vi "Actor Core.vi"(8 "error in":errorcluster, 11 "Stepper3D in":refnum<class "Stepper3D.lvclass">) -> (0 "error out":errorcluster, 3 "Actor  out":refnum<class "Actor.lvclass">)   [LabVIEW 2014, in "Stepper3D.lvclass"]
uses:
  Stepper3D.lvclass
  <vilib>/Utility/config.llb/NI_LVConfig.lvlib
  <vilib>/Utility/error.llb/DialogType.ctl
  Libs/array.lib/Array.lvlib
  Libs/stepper3D.lib/stepper3D.lvlib
  Libs/stepper3D.lib/Enums/BoundaryStatus.ctl
  <vilib>/Utility/config.llb/Read Key (Double).vi
  <vilib>/Utility/config.llb/Write Key (Double).vi
  Framework/Interfaces/Viewable Actor/Viewable Actor.lvclass
  Framework/Interfaces/Observable Actor/Observable Actor.lvclass
  Framework/Hardware/ParameterDevice/ParameterDevice.lvclass
  Stepper3D Messages/Set Conversion Table Msg/Set Conversion Table Msg.lvclass
  <vilib>/ActorFramework/Actor/Actor.lvclass
panel:
  in  "St3:DoSteps":bool
  in  "St2:DoSteps":bool
  out "WL:Real Value":dbl=450.0
  out "Stop":bool=TRUE
  out "St3:Right":bool
  out "St3:Left":bool
  out "St2:Right":bool
  out "St2:Left":bool
  out "St1:Right":bool
  out "St1:Left":bool
  in  "Speed":string="300"
  in  "UI:LoadConversionTables":bool
  in  "Conversion 3":path=path "C:/Users/219-PC/Dropbox/МФД/Alexandr Bogomolov/Кумарин 47/Эталон.txt"
  in  "Conversion 2":path=path "C:/Users/219-PC/Dropbox/МФД/Alexandr Bogomolov/Кумарин 47/Эталон.txt"
  in  "Conversion 1":path=path "C:/Users/219-PC/Dropbox/МФД/Alexandr Bogomolov/Кумарин 47/Кумарин 120.txt"
  out "WL:WLToStepper3":dbl[][](array[numeric])
  out "WL:WLToStepper2":dbl[][](array[numeric])=[[115.0, 0.0], [135.0, 0.0]]
  out "WL:WLToStepper1":dbl[][](array[numeric])
  in  "WL:NewValue":dbl=450.0
  in  "WL:Stop":bool
  in  "WL:SetValue":bool
  out "App:RefreshLED":bool
  in  "App:RefreshRate":u32=1000 caption="Refresh every"
  in  "App:Refresh":bool
  in  "App:Disconnect":bool
  in  "App:Connect":bool
  in  "St3:SetPos":bool
  in  "St2:SetPos":bool
  in  "St1:SetPos":bool
  in  "St:Stop":bool
  in  "St3:Steps":dbl
  in  "St3:NewPosition":dbl=2605.0
  out "St3:Position":dbl=2903.0
  in  "St2:Steps":dbl
  in  "St2:NewPosition":dbl=-2500.0
  out "St2:Position":dbl=-2500.0
  in  "St1:DoSteps":bool
  in  "St1:Steps":dbl
  in  "St1:NewPosition":dbl=-57680.0
  out "St1:Position":dbl=-57680.0
  in  "App:ResourceName":refnum<visa-resource-name>="COM8"
  # "ms."
  # "BOUNDARY"
  # "FUNCTIONS"
  # "POSITION"
  # "NEW POSITION"
  # "STEPS"
  # "Решетка"
  # "Фабри-Перо"
  # "Кристалл"
  # "Длина волны"
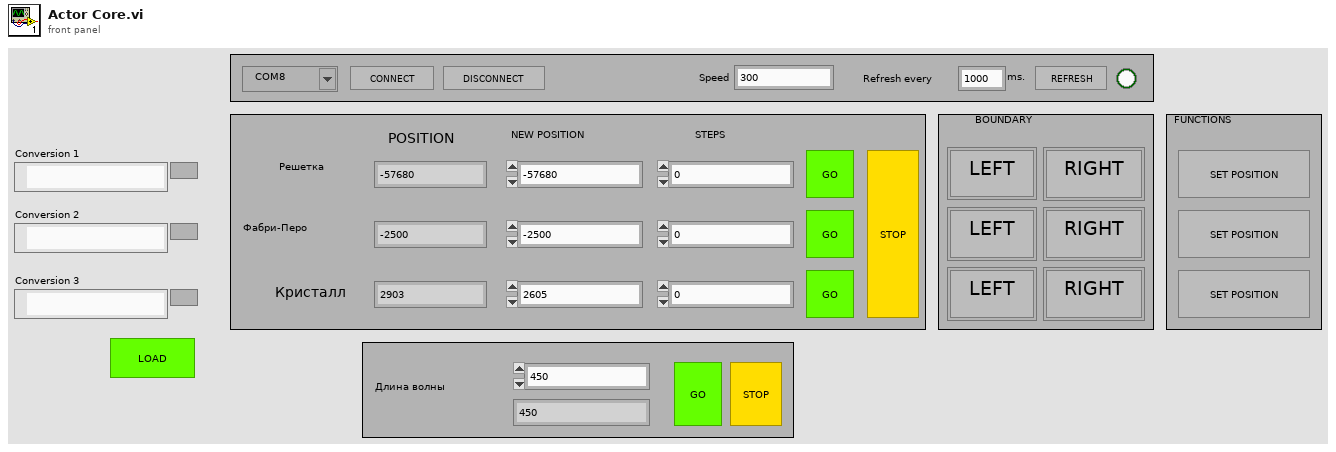
[diagram p1: front panel]
types:
  T1 = typedef "Observable Actor.lvlib/Observable Actor.lvclass/Observer.ctl" = refnum<queue>
  T2 = cluster{"steps":i32, "position":i32, "left":bool, "right":bool, "isRunning":bool, "stepper":u32}
  T3 = enum32{"invalid app kind", "Development System", "Run Time System", "Student Edition", "Embedded LabVIEW", "Evaluation", "Custom"}
  T4 = typedef "stepper3D.lvlib/BoundaryStatus.ctl" = enum16{"NO BOUNDARY", "OUT OF LEFT", "OUT OF RIGHT"}
  T5 = cluster{"Core":cluster{"Current VI Reference":refnum<vi>, "Close Panel on Exit?":bool}, "VISA resource":refnum<visa-resource-name>, "App:RefreshRate":u32, "isConnected":bool, "appended path":path}
  T6 = typedef "DialogType.ctl" = u16
  T7 = cluster{"Current VI Reference":refnum<vi>, "Close Panel on Exit?":bool}
  T8 = typedef "NI_LVConfig.lvlib/Config Data RefNum.ctl" = refnum<k1>
  T9 = enum8{"Enabled", "Disabled", "Disabled and Grayed Out"}
  T10 = typedef "stepper3D.lvlib/CurrentStatus.ctl" = cluster{"desired":dbl[], "current":dbl[], "boundaries":T4[], "is running":bool}
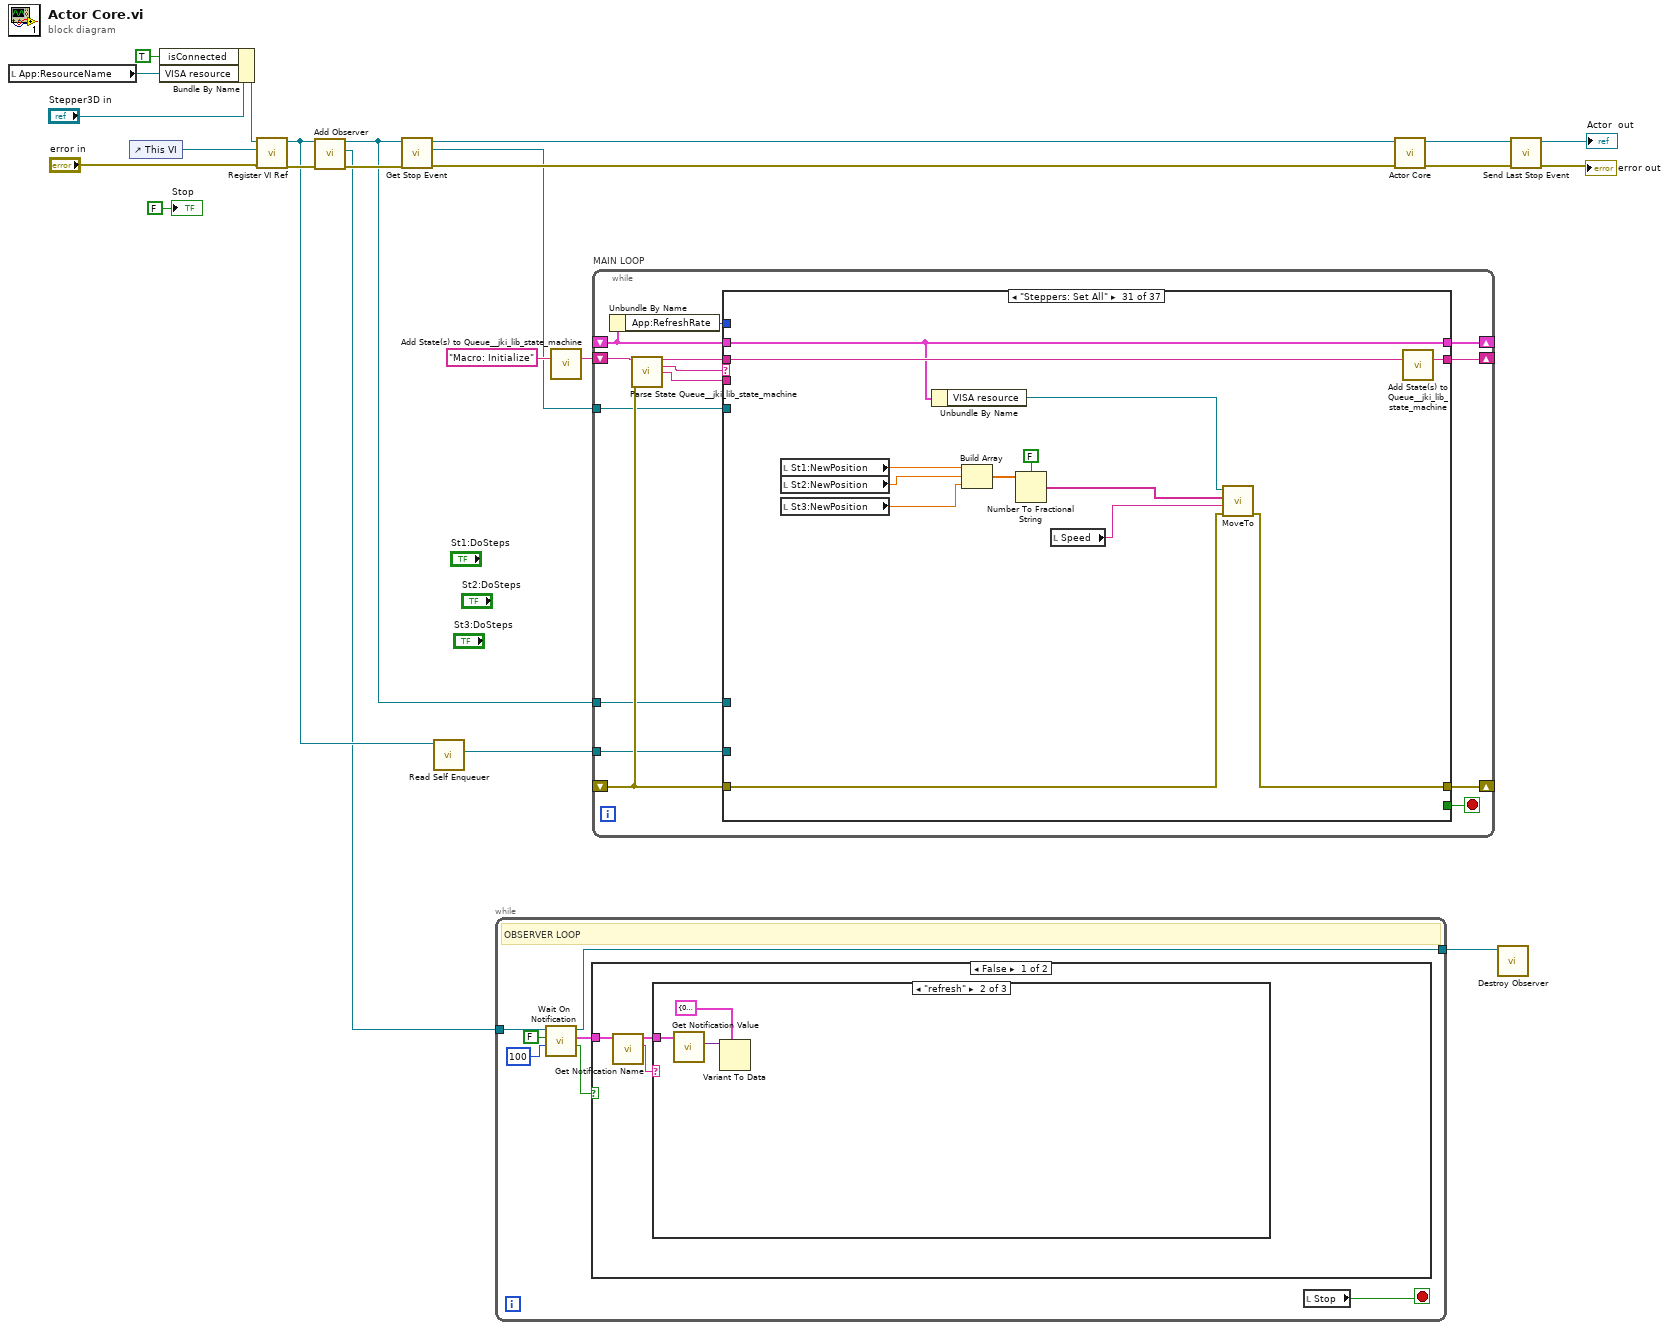
[diagram p0: block diagram]
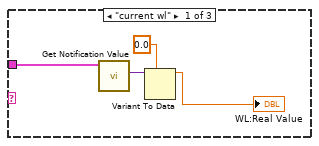
[diagram p2: hidden frame]
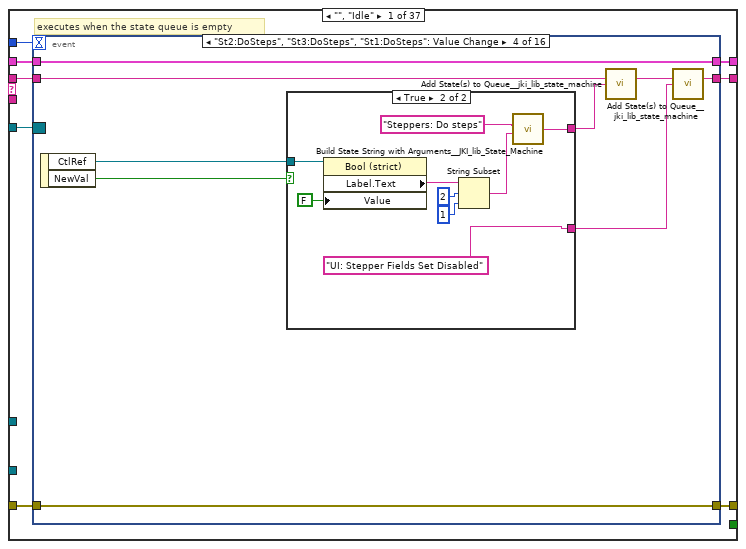
[diagram p5: hidden frame]
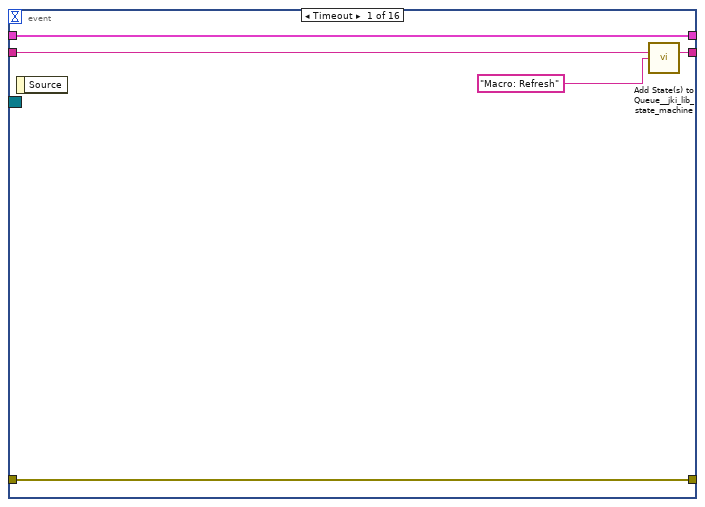
[diagram p6: hidden frame]
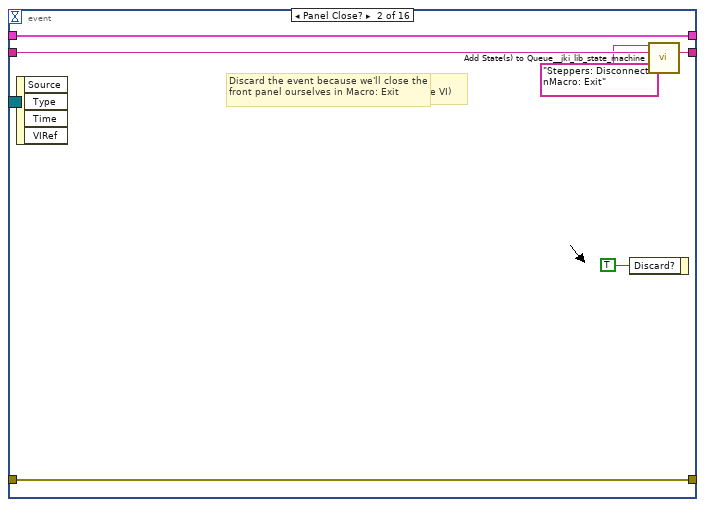
[diagram p7: hidden frame]
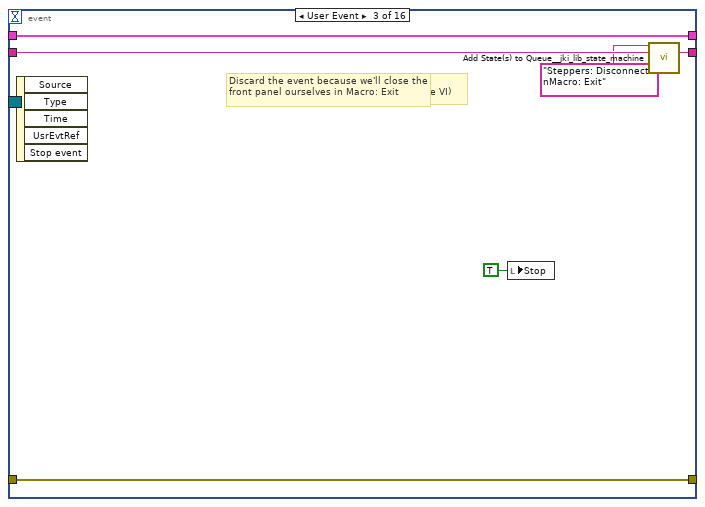
[diagram p8: hidden frame]
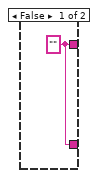
[diagram p9: hidden frame]
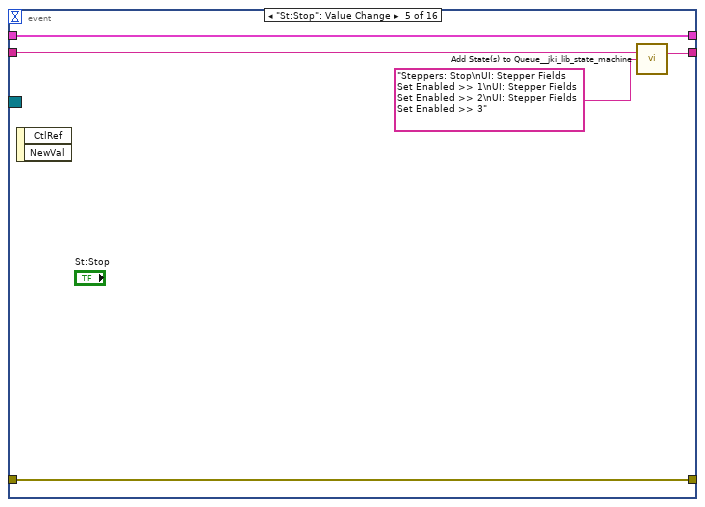
[diagram p10: hidden frame]
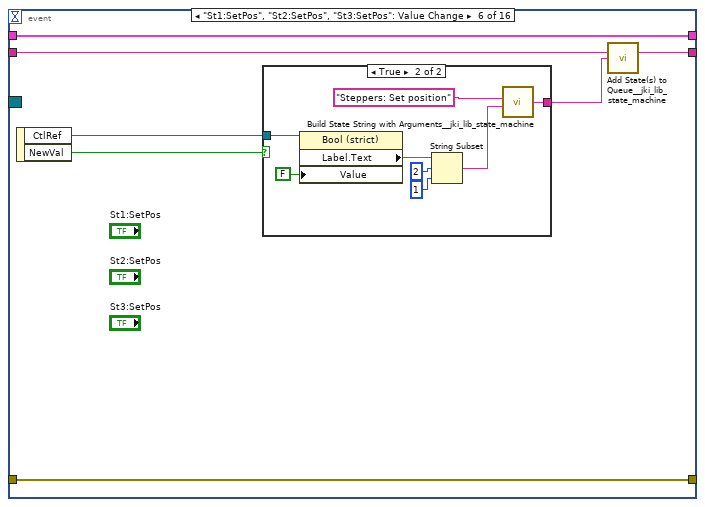
[diagram p11: hidden frame]
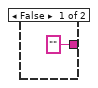
[diagram p12: hidden frame]
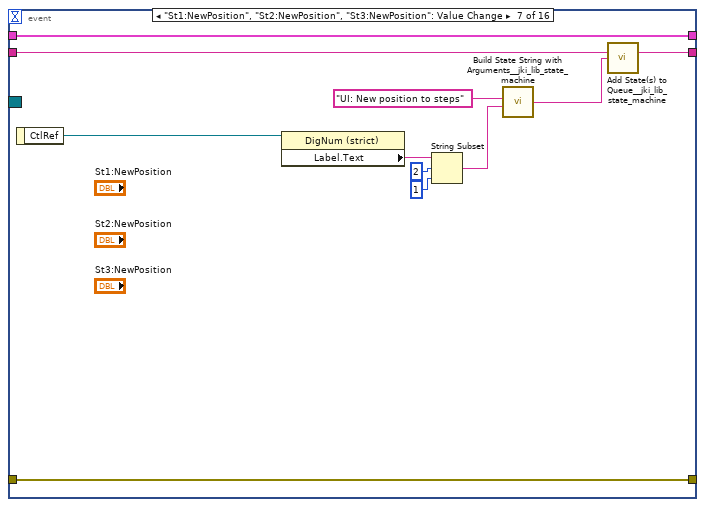
[diagram p13: hidden frame]
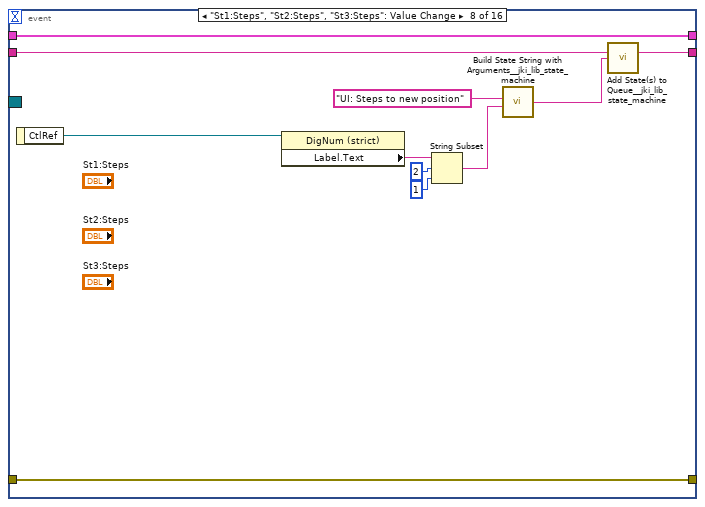
[diagram p14: hidden frame]
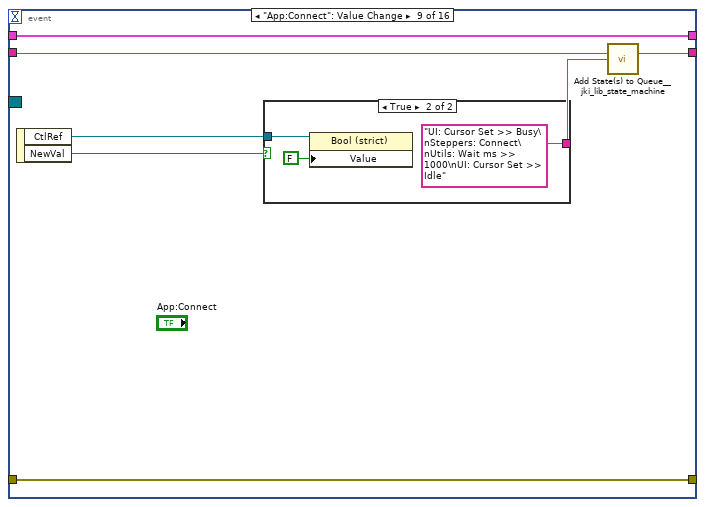
[diagram p15: hidden frame]
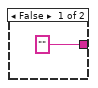
[diagram p16: hidden frame]
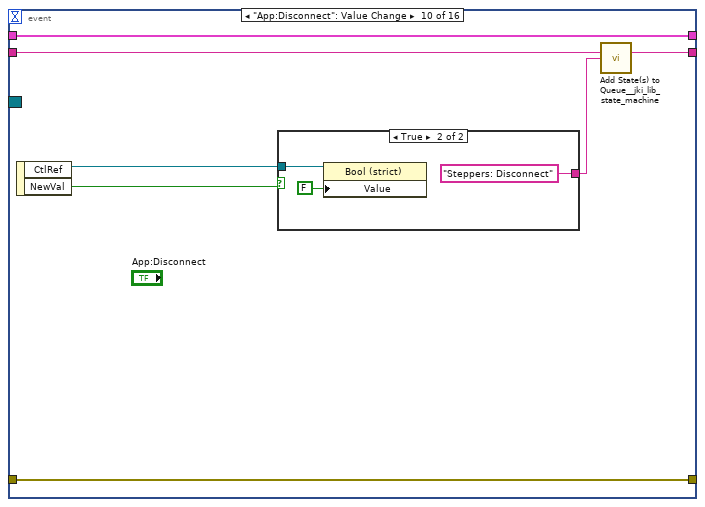
[diagram p17: hidden frame]
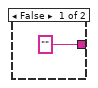
[diagram p18: hidden frame]
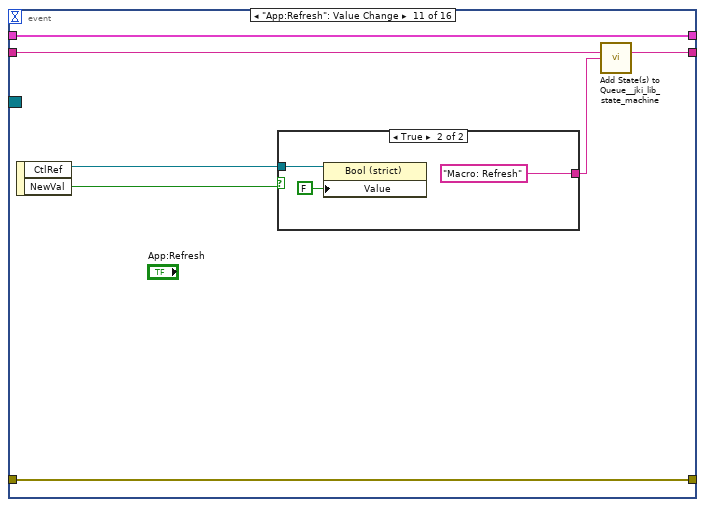
[diagram p19: hidden frame]
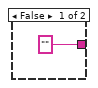
[diagram p20: hidden frame]
diagram:
  n1 = local read "App:ResourceName"() -> (w9:refnum<visa-resource-name>)
  n2 = control-ref of="This VI"() -> (w19:refnum<vi>)
  n3 = Bundle By Name(cluster="Stepper3D in", "isConnected"=TRUE, "VISA resource"=w9) -> (w11:refnum<class "Stepper3D.lvclass">)
  n4 = call "Register VI Ref.vi"("error in (no error)"="error in", "VI ref"=w19, "Viewable Actor in"=w11) -> ("error out"=w20:errorcluster, "Viewable Actor out"=w7:refnum<class "Stepper3D.lvclass">)  [unwired: 7 in]
  n5 = call-dynamic "Add Observer.vi"("error in (no error)"=w20, "Observable Actor in"=w7) -> ("error out"=w21:errorcluster, "new observer"=w2:T1, "Observable Actor out"=w1:refnum<class "Stepper3D.lvclass">)  [unwired: 7 in]
  n6 = call-dynamic "Get Stop Event.vi"("error in (no error)"=w21, "Observable Actor in"=w1) -> ("error out"=w14:errorcluster, "Events"=w8:refnum<event-registration>, "Observable Actor out"=w15:refnum<class "Stepper3D.lvclass">)  [unwired: 7 in]
  n7 = call <vilib>:"Read Self Enqueuer.vi"("Actor"=w7) -> ("Self Enqueuer"=w6:refnum<class "Message Enqueuer.lvclass">)  [unwired: 10 in]
  n8 = while {
    tunnel: w2 -> [w27]
    tunnel: [w26] -> w4
    stop <- w30 stop-if-true
    # "OBSERVER LOOP"
    n9 = call "Wait On Notification.vi"("timeout in ms (-1)"=100, "ignore previous (F)"=FALSE, "observer in"=w27) -> ("timed out?"=w24:bool, "notification"=w25:cluster{"value":variant, "name":string}, "observer out"=w26:T1)  [unwired: 5 in, 1 out]
    n10 = case shown="False" w24 {
      tunnel: w25 -> [w33 _]
      frame False {
        n11 = call "Get Notification Name.vi"("notification in"=w33) -> ("name"=w31:string, "notification out"=w32:cluster{"value":variant, "name":string})  [unwired: 9 in]
        n12 = case shown="\"refresh\"" w31 {
          tunnel: w32 -> [w35 w39 _]
          frame "current wl" {
            n13 = call "Get Notification Value.vi"("notification in"=w35) -> ("data"=w37:variant)  [unwired: 7 in, 1 out]
            n14 = Variant To Data(type=0.0 ("Current value"), Variant=w37) -> (data=→"WL:Real Value":dbl)  [unwired: 1 in, 1 out]
          }
          frame "refresh" {
            n15 = call "Get Notification Value.vi"("notification in"=w39) -> ("data"=w40:variant)  [unwired: 7 in, 1 out]
            n16 = Variant To Data(type=T2 {"steps"=0, "position"=0, "left"=FALSE, "right"=FALSE, "isRunning"=FALSE, "stepper"=0} ("input cluster"), Variant=w40) -> ()  [unwired: 1 in, 2 out]
          }
          frame Default {
          }
        }
      }
      frame True {
      }
    }
    n17 = local read "Stop"() -> (w30:bool)
  }
  n18 = call <vilib>:"Add State(s) to Queue__jki_lib_state_machine.vi"("State(s) in (\"\")"="Macro: Initialize") -> ("States Out"=w23:string)  [unwired: 14 in]
  n19 = while "MAIN LOOP" {
    shift-right: [w48] -> _
    shift-left: _ -> [w44]
    shift-right: [w51] -> _
    shift-left: _ -> [w47]
    shift-right: [w50] -> _
    shift-left: w23 -> [w52]
    tunnel: w8 -> [w43]
    tunnel: w6 -> [w42]
    tunnel: w1 -> [w41]
    stop <- w49 stop-if-true
    n20 = Unbundle By Name(w44) -> ("App:RefreshRate"=w45:u32)
    n21 = call <vilib>:"Parse State Queue__jki_lib_state_machine.vi"("State Queue"=w52, "Error In (no error)"=w47) -> ("Remaining States"=w54:string, "Current State"=w46:string, "Arguments"=w53:string)  [unwired: 11 in]
    n22 = case shown="\"Steppers: Set All\"" w46 {
      selector: w46 -> [_ _ w215 _ _ _ _ _ _ _ _ _ _ _ _ _ _ _ _ _ _ _ _ _ _ _ _ _ _ _ _ _ _ _ _ _ _]
      tunnel: w54 -> [w62 w214 w219 w237 w244 w249 w253 w268 w279 w298 w320 w326 w330 w335 w340 w345 w347 w366 w369 w385 w386 w394 w399 w404 w410 w422 w426 w434 w441 w460 w477 w494 w505 w508 w576 w581 w588]
      tunnel: w53 -> [_ _ _ _ _ _ _ _ _ _ _ _ _ _ _ _ w346 _ w370 _ w389 _ _ _ _ _ _ _ _ w450 _ w490 _ _ _ _ w584]
      tunnel: w44 -> [w60 w211 w217 w228 w241 w247 w250 w265 _ w296 w317 w322 w327 w332 w337 w343 w349 w368 w372 w383 w390 w395 w396 w401 w407 w419 w423 w437 w440 w458 w475 w491 w503 w513 w577 w578 w585]
      tunnel: [w59 w212 w221 w234 errorcluster {"status"=FALSE, "code"=0, "source"=""} ("error out") w246 w251 w266 w276 w280 w318 w323 w328 w333 w338 w342 w348 w367 w371 w382 w388 w393 w397 w402 w408 w420 w424 w427 w442 w455 w472 w489 w500 w510 w572 w579 w586] -> w51
      tunnel: w47 -> [w58 w212 w220 w234 w240 w246 w251 w266 w276 w281 w318 w321 w328 w333 w338 w342 w348 w367 w371 w382 w388 w393 w397 w402 w408 w420 w424 w428 w443 w456 w473 w488 w501 w511 w573 w579 w586]
      tunnel: [w61 w213 w218 w236 w243 w248 w252 w267 w278 w297 w319 w325 w329 w334 w339 w344 w347 w366 w369 w384 w386 w394 w398 w403 w409 w421 w425 w435 w441 w459 w476 w493 w504 w507 w575 w580 w587] -> w50
      tunnel: [_ _ _ _ _ TRUE _ _ _ _ _ _ _ _ _ _ _ _ _ _ _ _ _ _ _ _ _ _ _ _ _ _ _ _ _ _ _] -> w49
      tunnel: [w57 w211 w217 w235 w241 w247 w250 w265 w277 w296 w317 w322 w327 w332 w337 w343 w349 w368 w372 w383 w390 w395 w396 w401 w407 w419 w423 w436 w439 w458 w475 w491 w503 w513 w577 w578 w585] -> w48
      tunnel: w45 -> [w56 _ _ _ _ _ _ _ _ _ _ _ _ _ _ _ _ _ _ _ _ _ _ _ _ _ _ _ _ _ _ _ _ _ _ _ _]
      tunnel: w43 -> [w55 _ _ _ _ _ _ _ _ _ _ _ _ _ _ _ _ _ _ _ _ _ _ _ _ _ _ _ _ _ _ _ _ _ _ _ _]
      tunnel: w42 -> [_ _ _ _ _ _ _ w257 _ _ _ _ _ _ _ _ _ _ _ _ _ _ _ _ _ _ _ _ _ _ _ _ _ _ _ _ _]
      tunnel: w41 -> [_ _ _ _ _ _ _ _ _ _ _ _ _ _ _ _ _ _ _ _ _ _ _ _ _ _ _ _ _ _ _ _ _ _ w574 _ _]
      frame "", "Idle" {
        # "executes when the state queue is empty"
        n23 = event shown="[3] \"St2:DoSteps\", \"St3:DoSteps\", \"St1:DoSteps\": Value Change" {
          selector: w55 -> [_ _ _ _ _ _ _ _ _ _ _ _ _ _ _ _]
          dyn-events: _ -> [_ _ _ _ _ _ _ _ _ _ _ _ _ _ _ _]
          timeout: w56 -> [_ _ _ _ _ _ _ _ _ _ _ _ _ _ _ _]
          tunnel: w62 -> [w67 w73 w79 w84 w100 w106 w127 w138 w145 w155 w166 w180 w185 w191 w199 w207]
          tunnel: [w66 w72 w78 w82 w101 w105 w126 w137 w146 w156 w167 w181 w186 w192 w200 w208] -> w61
          tunnel: w60 -> [w64 w70 w76 w87 w103 w109 w129 w140 w147 w159 w170 w177 w183 w189 w197 w205]
          tunnel: [w65 w71 w77 w86 w102 w108 w128 w139 w148 w153 w164 w178 w184 w190 w198 w206] -> w59
          tunnel: w58 -> [w65 w71 w77 w86 w102 w108 w128 w139 w148 w153 w164 w178 w184 w190 w198 w206]
          tunnel: [w64 w70 w76 w87 w103 w109 w129 w140 w147 w159 w170 w176 w183 w189 w197 w205] -> w57
          event Timeout {
            n24 = event-data() -> ()  [unwired: 1 in, 1 out]
            n25 = call <vilib>:"Add State(s) to Queue__jki_lib_state_machine.vi"("State(s) in (\"\")"=w67, "State(s) at Back (\"\")"="Macro: Refresh") -> ("States Out"=w66:string)  [unwired: 13 in]
          }
          event Panel Close? {
            # "Discard the event because we'll close the front panel ourselves in Macro: Exit"
            # "Close Panel button (pressed) Event\n(this executes Macro: Exit to terminate the VI)"
            n26 = event-data() -> ()  [unwired: 1 in, 4 out]
            n27 = event-data("Discard?"=TRUE) -> ()  [unwired: 1 in, 1 out]
            n28 = call <vilib>:"Add State(s) to Queue__jki_lib_state_machine.vi"("State(s) in Front (\"\")"="Steppers: Disconnect\nMacro: Exit", "State(s) in (\"\")"=w73) -> ("States Out"=w72:string)  [unwired: 13 in]
          }
          event User Event {
            # "Discard the event because we'll close the front panel ourselves in Macro: Exit"
            # "Close Panel button (pressed) Event\n(this executes Macro: Exit to terminate the VI)"
            n29 = event-data() -> ()  [unwired: 1 in, 5 out]
            n30 = local write "Stop"(TRUE ("Stop")) -> ()
            n31 = call <vilib>:"Add State(s) to Queue__jki_lib_state_machine.vi"("State(s) in Front (\"\")"="Steppers: Disconnect\nMacro: Exit", "State(s) in (\"\")"=w79) -> ("States Out"=w78:string)  [unwired: 13 in]
          }
          event "St2:DoSteps", "St3:DoSteps", "St1:DoSteps": Value Change {
            n32 = event-data() -> ("CtlRef"=w88:refnum<vi>, "NewVal"=w85:bool)  [unwired: 1 in]
            n33 = case shown="True" w85 {
              tunnel: w88 -> [_ w98]
              tunnel: [w89 w94] -> w83
              tunnel: [w89 "UI: Stepper Fields Set Disabled" ("State")] -> w80
              frame False {
                w89 = "" ("State with Arguments")
              }
              frame True {
                n34 = property class="Bool (strict)"(reference=w98, "Value"=FALSE) -> ("Label.Text"=w91:string)  [unwired: 1 in, 2 out]
                n35 = String Subset(string=w91, offset (0)=2, length (rest)=1 ("length (rest)")) -> (substring=w90:string)
                n36 = call <vilib>:"Build State String with Arguments__JKI_lib_State_Machine.vi"("Arguments (\"\")"=w90, "State"="Steppers: Do steps") -> ("State with Arguments"=w94:string)  [unwired: 4 in]
              }
            }
            n37 = call <vilib>:"Add State(s) to Queue__jki_lib_state_machine.vi"("State(s) in (\"\")"=w84, "State(s) at Back (\"\")"=w83) -> ("States Out"=w81:string)  [unwired: 13 in]
            n38 = call <vilib>:"Add State(s) to Queue__jki_lib_state_machine.vi"("State(s) in (\"\")"=w81, "State(s) at Back (\"\")"=w80) -> ("States Out"=w82:string)  [unwired: 13 in]
          }
          event "St:Stop": Value Change {
            n39 = event-data() -> ()  [unwired: 1 in, 2 out]
            n40 = call <vilib>:"Add State(s) to Queue__jki_lib_state_machine.vi"("State(s) in (\"\")"=w100, "State(s) at Back (\"\")"="Steppers: Stop\nUI: Stepper Fields Set Enabled >> 1\nUI: Stepper Fields Set Enabled >> 2\nUI: Stepper Fields Set Enabled >> 3" ("State")) -> ("States Out"=w101:string)  [unwired: 13 in]
          }
          event "St1:SetPos", "St2:SetPos", "St3:SetPos": Value Change {
            n41 = event-data() -> ("CtlRef"=w110:refnum<vi>, "NewVal"=w107:bool)  [unwired: 1 in]
            n42 = case shown="True" w107 {
              tunnel: w110 -> [_ w119]
              tunnel: ["" ("State with Arguments") w113] -> w104
              frame False {
              }
              frame True {
                n43 = property class="Bool (strict)"(reference=w119, "Value"=FALSE) -> ("Label.Text"=w116:string)  [unwired: 1 in, 2 out]
                n44 = String Subset(string=w116, offset (0)=2, length (rest)=1 ("length (rest)")) -> (substring=w114:string)
                n45 = call <vilib>:"Build State String with Arguments__jki_lib_state_machine.vi"("Arguments (\"\")"=w114, "State"="Steppers: Set position") -> ("State with Arguments"=w113:string)  [unwired: 4 in]
              }
            }
            n46 = call <vilib>:"Add State(s) to Queue__jki_lib_state_machine.vi"("State(s) in (\"\")"=w106, "State(s) at Back (\"\")"=w104) -> ("States Out"=w105:string)  [unwired: 13 in]
          }
          event "St1:NewPosition", "St2:NewPosition", "St3:NewPosition": Value Change {
            n47 = event-data() -> ("CtlRef"=w130:refnum<vi>)  [unwired: 1 in]
            n48 = property class="DigNum (strict)"(reference=w130) -> ("Label.Text"=w122:string)  [unwired: 1 in, 2 out]
            n49 = String Subset(string=w122, offset (0)=2, length (rest)=1 ("length (rest)")) -> (substring=w120:string)
            n50 = call <vilib>:"Build State String with Arguments__jki_lib_state_machine.vi"("Arguments (\"\")"=w120, "State"="UI: New position to steps") -> ("State with Arguments"=w125:string)  [unwired: 4 in]
            n51 = call <vilib>:"Add State(s) to Queue__jki_lib_state_machine.vi"("State(s) in (\"\")"=w127, "State(s) at Back (\"\")"=w125) -> ("States Out"=w126:string)  [unwired: 13 in]
          }
          event "St1:Steps", "St2:Steps", "St3:Steps": Value Change {
            n52 = event-data() -> ("CtlRef"=w141:refnum<vi>)  [unwired: 1 in]
            n53 = property class="DigNum (strict)"(reference=w141) -> ("Label.Text"=w133:string)  [unwired: 1 in, 2 out]
            n54 = String Subset(string=w133, offset (0)=2, length (rest)=1 ("length (rest)")) -> (substring=w131:string)
            n55 = call <vilib>:"Build State String with Arguments__jki_lib_state_machine.vi"("Arguments (\"\")"=w131, "State"="UI: Steps to new position") -> ("State with Arguments"=w136:string)  [unwired: 4 in]
            n56 = call <vilib>:"Add State(s) to Queue__jki_lib_state_machine.vi"("State(s) in (\"\")"=w138, "State(s) at Back (\"\")"=w136) -> ("States Out"=w137:string)  [unwired: 13 in]
          }
          event "App:Connect": Value Change {
            n57 = event-data() -> ("CtlRef"=w144:refnum<vi>, "NewVal"=w143:bool)  [unwired: 1 in]
            n58 = case shown="True" w143 {
              tunnel: w144 -> [_ w152]
              tunnel: ["" "UI: Cursor Set >> Busy\nSteppers: Connect\nUtils: Wait ms >> 1000\nUI: Cursor Set >> Idle"] -> w142
              frame False {
              }
              frame True {
                n59 = property class="Bool (strict)"(reference=w152, "Value"=FALSE) -> ()  [unwired: 1 in, 2 out]
              }
            }
            n60 = call <vilib>:"Add State(s) to Queue__jki_lib_state_machine.vi"("State(s) in (\"\")"=w145, "State(s) at Back (\"\")"=w142) -> ("States Out"=w146:string)  [unwired: 13 in]
          }
          event "App:Disconnect": Value Change {
            n61 = event-data() -> ("CtlRef"=w158:refnum<vi>, "NewVal"=w157:bool)  [unwired: 1 in]
            n62 = case shown="True" w157 {
              tunnel: w158 -> [_ w163]
              tunnel: ["" "Steppers: Disconnect"] -> w154
              frame False {
              }
              frame True {
                n63 = property class="Bool (strict)"(reference=w163, "Value"=FALSE) -> ()  [unwired: 1 in, 2 out]
              }
            }
            n64 = call <vilib>:"Add State(s) to Queue__jki_lib_state_machine.vi"("State(s) in (\"\")"=w155, "State(s) at Back (\"\")"=w154) -> ("States Out"=w156:string)  [unwired: 13 in]
          }
          event "App:Refresh": Value Change {
            n65 = event-data() -> ("CtlRef"=w169:refnum<vi>, "NewVal"=w168:bool)  [unwired: 1 in]
            n66 = case shown="True" w168 {
              tunnel: w169 -> [_ w174]
              tunnel: ["" "Macro: Refresh"] -> w165
              frame False {
              }
              frame True {
                n67 = property class="Bool (strict)"(reference=w174, "Value"=FALSE) -> ()  [unwired: 1 in, 2 out]
              }
            }
            n68 = call <vilib>:"Add State(s) to Queue__jki_lib_state_machine.vi"("State(s) in (\"\")"=w166, "State(s) at Back (\"\")"=w165) -> ("States Out"=w167:string)  [unwired: 13 in]
          }
          event "App:RefreshRate": Value Change {
            n69 = event-data() -> ()  [unwired: 1 in, 1 out]
            n70 = Bundle By Name(cluster=w177, "App:RefreshRate"="App:RefreshRate") -> (w176:T5)
            n71 = call <vilib>:"Add State(s) to Queue__jki_lib_state_machine.vi"("State(s) in (\"\")"=w180, "State(s) at Back (\"\")"="Steppers: Set refresh rate") -> ("States Out"=w181:string)  [unwired: 13 in]
          }
          event "WL:NewValue": Value Change {
            n72 = event-data() -> ()  [unwired: 1 in, 6 out]
            n73 = call <vilib>:"Add State(s) to Queue__jki_lib_state_machine.vi"("State(s) in (\"\")"=w185, "State(s) at Back (\"\")"="UI: New WL to positions" ("State(s) at Back (\"\")")) -> ("States Out"=w186:string)  [unwired: 13 in]
          }
          event "WL:SetValue": Value Change {
            n74 = event-data() -> ("NewVal"=w188:bool)  [unwired: 1 in]
            n75 = case shown="False" w188 {
              tunnel: ["" "Steppers: Set All"] -> w187
              frame False {
              }
              frame True {
                n76 = property on="WL:SetValue" class="Bool (strict)"("Value"=FALSE ("WL:SetValue")) -> ()  [unwired: 2 in, 2 out]
              }
            }
            n77 = call <vilib>:"Add State(s) to Queue__jki_lib_state_machine.vi"("State(s) in (\"\")"=w191, "State(s) at Back (\"\")"=w187) -> ("States Out"=w192:string)  [unwired: 13 in]
          }
          event "WL:Stop": Value Change {
            n78 = event-data() -> ("NewVal"=w196:bool)  [unwired: 1 in]
            n79 = case shown="True" w196 {
              frame False {
              }
              frame True {
                n80 = property on="WL:Stop" class="Bool (strict)"("Value"=FALSE ("WL:Stop")) -> ()  [unwired: 2 in, 2 out]
                n81 = property on="St:Stop" class="Bool (strict)"("Val(Sgnl)"=TRUE) -> ()  [unwired: 2 in, 2 out]
              }
            }
            n82 = call <vilib>:"Add State(s) to Queue__jki_lib_state_machine.vi"("State(s) in (\"\")"=w199) -> ("States Out"=w200:string)  [unwired: 14 in]
          }
          event "UI:LoadConversionTables": Value Change {
            n83 = event-data() -> ("NewVal"=w204:bool)  [unwired: 1 in]
            n84 = case shown="True" w204 {
              tunnel: [_ "Data: Load Conversion Files"] -> w203
              frame False {
              }
              frame True {
                n85 = property on="UI:LoadConversionTables" class="Bool (strict)"("Value"=FALSE) -> ()  [unwired: 2 in, 2 out]
              }
            }
            n86 = call <vilib>:"Add State(s) to Queue__jki_lib_state_machine.vi"("State(s) in (\"\")"=w207, "State(s) at Back (\"\")"=w203) -> ("States Out"=w208:string)  [unwired: 13 in]
          }
        }
      }
      frame "---------- Core ----------" {
        # "Do not put any code in this frame.\n(it is a separator no-op)"
        n87 = call <vilib>:"Add State(s) to Queue__jki_lib_state_machine.vi"("State(s) in (\"\")"=w214) -> ("States Out"=w213:string)  [unwired: 14 in]
      }
      frame Default {
        w224 = 42 items=["No error", "Argument error", "Memory is full", "Out of zone", "End of file", "File already open", "Generic file I/O error", "File not found", "File permission error", "Disk is full", "Duplicate path", "Too many files open", "System feature not enabled", "Resource file not found", "Cannot add resource", "Resource not found", "Image not found", "Image memory error", "Pen does not exist", "Config type invalid", "Config token not found", "Config parse error", "Config memory error", "Bad external code format", "Bad external code offset", "External code not present", "Null window", "Destroy window error", "Null menu", "Print aborted", "Bad print record", "Print driver error", "Windows error during printing", "Memory error during printing", "Print dialog error", "Generic print error", "Invalid device refnum", "Device not found", "Device parameter error", "Device unit error", "Cannot open device", "Device call aborted", "Generic error", "Cancelled by user", "Object ID too low", "Object ID too high", "Object not in heap", "Unknown heap", "Unknown object (invalid DefProc)", "Unknown object (DefProc not in table)", "Message out of range", "Invalid (null) method", "Unknown message", "Manager call not supported", "Bad address", "Network operation in progress", "Network operation timed out", "Connection is busy", "Network attribute not supported", "Network error", "Address in use", "System out of memory", "Connection aborted", "Connection refused", "Not connected", "Already connected", "Connection closed", "Initialization error (interapplication manager)", "Bad occurrence", "Wait on unbound occurrence handler", "Occurrence queue overflow", "Datalog type conflict", "Unused", "Unrecognized type (interapplication manager)", "Memory corrupt", "Failed to make temporary DLL", "Old CIN version", "Drag socket not found", "Failed to load drop-object", "Failed to register OLE object", "Failed to release OLE object", "Format specifier type mismatch", "Unknown format specifier", "Too few format specifiers", "Too many format specifiers", "Scan failed", "Newer CIN version", "Error converting to variant", "Runtime menu error", "Password tampered", "Variant attribute not found", "Incompatible variant data type", "Event data is not available", "Event Store is not present", "Occurrence is not found", "Event Queue is not created", "Event info is not available", "Refnum passed is NULL", "Error retrieving Class GUID", "Error retrieving CoClass GUID", "Error retrieving TypeLib GUID.", "Bad built application magic bytes.", "Specific driver is different from the specific driver associated with the Logical Name.", "There is no session opened to the class driver.", "Max Error", "MAX - Error with config objects", "MAX - Error loading configuration", "MAX - Group not supported"]
        # "Current State"
        # "Handle mistyped state name (developer tool)"
        n88 = Format Into String(format string="Software Exception: Unhandled State \"%s\"." ("message"), error in=w220, w215) -> (resulting string=w223:string, error out=w222:errorcluster)  [unwired: 1 in]
        n89 = call <vilib>:"Error Cluster From Error Code.vi"("show call chain? (False)"=TRUE, "error in (no error)"=w222, "error message (\"\")"=w223, "error code (0)"=w224) -> ("error out"=w221:errorcluster)  [unwired: 5 in]
        n90 = call <vilib>:"Add State(s) to Queue__jki_lib_state_machine.vi"("State(s) in (\"\")"=w219) -> ("States Out"=w218:string)  [unwired: 14 in]
      }
      frame "Initialize Core Data" {
        # "originally closed?"
        # "exe?"
        # "If panel starts closed or is an EXE, then close it when we exit"
        n91 = property class="VI"() -> ("Front Panel.Open"=w233:bool)  [unwired: 2 in, 2 out]
        n92 = property class="App"() -> ("App.Kind"=w232:T3)  [unwired: 2 in, 2 out]
        n93 = control-ref of="Current VI Reference"() -> (w226:refnum<vi>)
        n94 = Not(x=w233) -> (.not. x?=w230:bool)
        n95 = Equal?(x=w232, y=T3."Run Time System" ("Application:Kind")) -> (x = y?=w229:bool)
        n96 = Or(x=w230, y=w229) -> (x .or. y?=w227:bool)
        n97 = Bundle By Name(cluster=w228, "Core.Current VI Reference"=w226, "Core.Close Panel on Exit?"=w227) -> (w235:T5)
        n98 = call <vilib>:"Add State(s) to Queue__jki_lib_state_machine.vi"("State(s) in (\"\")"=w237) -> ("States Out"=w236:string)  [unwired: 14 in]
      }
      frame "Error Handler" {
        w238 = T6 2 items=["no dialog", "OK message", "continue or stop message", "OK message + warnings", "continue/stop + warnings"] ("type of dialog (OK msg:1)")
        # "Unhandled Error -- Display it"
        # "Handle any errors here.\nYou can also output any states to clean-up after errors occur"
        # "Clear error"
        n99 = call <vilib>:"General Error Handler.vi"("type of dialog (OK msg:1)"=w238, "error in (no error)"=w240) -> ()  [unwired: 9 in, 5 out]
        n100 = call <vilib>:"Add State(s) to Queue__jki_lib_state_machine.vi"("State(s) in Front (\"\")"="// Post Error States", "State(s) in (\"\")"=w244) -> ("States Out"=w243:string)  [unwired: 13 in]
      }
      frame "Exit" {
        n101 = call <vilib>:"Add State(s) to Queue__jki_lib_state_machine.vi"("State(s) in (\"\")"=w249) -> ("States Out"=w248:string)  [unwired: 14 in]
      }
      frame "---------- Data ----------" {
        # "Do not put any code in this frame.\n(It is a separator no-op. You can make a copy of this frame to create a new Data frame)"
        n102 = call <vilib>:"Add State(s) to Queue__jki_lib_state_machine.vi"("State(s) in (\"\")"=w253) -> ("States Out"=w252:string)  [unwired: 14 in]
      }
      frame "Data: Load Conversion Files" {
        n103 = call "readArrayFromFile.vi"("file"="Conversion 1") -> ("array"=w256:dbl[][])  [unwired: 1 in, 1 out]
        "WL:WLToStepper1" <- w256
        n104 = call "readArrayFromFile.vi"("file"="Conversion 2") -> ("array"=w255:dbl[][])  [unwired: 1 in, 1 out]
        "WL:WLToStepper2" <- w255
        n105 = call "readArrayFromFile.vi"("file"="Conversion 3") -> ("array"=w254:dbl[][])  [unwired: 1 in, 1 out]
        "WL:WLToStepper3" <- w254
        n106 = call "Send Set Conversion Table.vi"("Stepper"=u32 1, "Conversion table"=w256, "Message Enqueuer"=w257) -> ()  [unwired: 7 in, 2 out]
        n107 = call "Send Set Conversion Table.vi"("Stepper"=u32 2, "Conversion table"=w255, "Message Enqueuer"=w257) -> ()  [unwired: 7 in, 2 out]
        n108 = call "Send Set Conversion Table.vi"("Stepper"=u32 3, "Conversion table"=w254, "Message Enqueuer"=w257) -> ()  [unwired: 7 in, 2 out]
        n109 = call <vilib>:"Add State(s) to Queue__jki_lib_state_machine.vi"("State(s) in (\"\")"=w268, "State(s) at Back (\"\")"="UI: New WL to positions" ("State(s) at Back (\"\")")) -> ("States Out"=w267:string)  [unwired: 13 in]
      }
      frame "Data: Initialize" {
        w273 = FALSE  # isConnected
        w274 = refnum<visa-resource-name> refnum  # VISA resource
        w275 = T7 {"Current VI Reference"=refnum, "Close Panel on Exit?"=FALSE}  # Core
        n110 = local read "App:RefreshRate"() -> (w272:u32)
        n111 = call <vilib>:"Application Directory.vi"() -> ("Application Directory"=w271:path)
        n112 = Build Path(base path=w271, name or relative path="steppers.config") -> (appended path=w269:path)
        n113 = Bundle("Core"=w275, "VISA resource"=w274, "App:RefreshRate"=w272, "isConnected"=w273, "appended path"=w269) -> (w277:T5)  [unwired: 1 in]
        n114 = call <vilib>:"Add State(s) to Queue__jki_lib_state_machine.vi"("State(s) in (\"\")"=w279) -> ("States Out"=w278:string)  [unwired: 14 in]
      }
      frame "Data: Read Config" {
        n115 = Unbundle By Name(w296) -> ("appended path"=w283:path)
        n116 = call <vilib>:"Open Config Data.vi"("error in (no error)"=w281, "configuration file path"=w283) -> ("error out"=w280:errorcluster, "refnum"=w282:T8)  [unwired: 7 in, 1 out]
        n117 = call-poly <vilib>:"Read Key.vi"("section"="current values", "key"="wavelength", "refnum"=w282) -> ("value"=w287:dbl)  [unwired: 5 in, 3 out]
        n118 = call-poly <vilib>:"Read Key.vi"("section"="current values", "key"="stepper1", "refnum"=w282) -> ("value"=w286:dbl)  [unwired: 5 in, 3 out]
        n119 = call-poly <vilib>:"Read Key.vi"("section"="current values", "key"="stepper2", "refnum"=w282) -> ("value"=w285:dbl)  [unwired: 5 in, 3 out]
        n120 = call-poly <vilib>:"Read Key.vi"("section"="current values", "key"="stepper3", "refnum"=w282) -> ("value"=w284:dbl)  [unwired: 5 in, 3 out]
        n121 = local write "WL:NewValue"(w287) -> ()
        n122 = local write "St1:NewPosition"(w286) -> ()
        n123 = local write "St2:NewPosition"(w285) -> ()
        n124 = local write "St3:NewPosition"(w284) -> ()
        n125 = call <vilib>:"Add State(s) to Queue__jki_lib_state_machine.vi"("State(s) in (\"\")"=w298) -> ("States Out"=w297:string)  [unwired: 14 in]
      }
      frame "Data: Write Config" {
        n126 = Unbundle By Name(w317) -> ("appended path"=w301:path)
        n127 = local read "St1:Position"() -> (w307:dbl)
        n128 = local read "WL:NewValue"() -> (w308:dbl)
        n129 = local read "St2:Position"() -> (w306:dbl)
        n130 = local read "St3:Position"() -> (w305:dbl)
        n131 = call <vilib>:"Open Config Data.vi"("configuration file path"=w301) -> ("refnum"=w300:T8)  [unwired: 8 in, 2 out]
        n132 = call-poly <vilib>:"Write Key.vi"("section"="current values", "value"=w308, "key"="wavelength", "refnum"=w300) -> ("refnum out"=w304:T8)  [unwired: 5 in, 2 out]
        n133 = call-poly <vilib>:"Write Key.vi"("section"="current values", "value"=w307, "key"="stepper1", "refnum"=w304) -> ("refnum out"=w303:T8)  [unwired: 5 in, 2 out]
        n134 = call-poly <vilib>:"Write Key.vi"("section"="current values", "value"=w306, "key"="stepper2", "refnum"=w303) -> ("refnum out"=w302:T8)  [unwired: 5 in, 2 out]
        n135 = call-poly <vilib>:"Write Key.vi"("section"="current values", "value"=w305, "key"="stepper3", "refnum"=w302) -> ("refnum out"=w299:T8)  [unwired: 5 in, 2 out]
        n136 = call <vilib>:"Close Config Data.vi"("refnum"=w299) -> ()  [unwired: 9 in, 2 out]
        n137 = call <vilib>:"Add State(s) to Queue__jki_lib_state_machine.vi"("State(s) in (\"\")"=w320) -> ("States Out"=w319:string)  [unwired: 14 in]
      }
      frame "Data: Cleanup" {
        n138 = Unbundle By Name(w322) -> ("Core.Current VI Reference"=w324:refnum<vi>)
        n139 = Close Reference(reference=w324, error in (no error)=w321) -> (error out=w323:errorcluster)
        n140 = call <vilib>:"Add State(s) to Queue__jki_lib_state_machine.vi"("State(s) in (\"\")"=w326) -> ("States Out"=w325:string)  [unwired: 14 in]
      }
      frame "---------- UI ----------" {
        # "Do not put any code in this frame.\n(It is a separator no-op. You can make a copy of this frame to create a new UI frame)"
        n141 = call <vilib>:"Add State(s) to Queue__jki_lib_state_machine.vi"("State(s) in (\"\")"=w330) -> ("States Out"=w329:string)  [unwired: 14 in]
      }
      frame "UI: Stepper Fields Set Enabled" {
        w331 = T9."Enabled" ("Disabled")
        # "Set Stepper Fields state .\n(Usage: \"UI: Stepper Fields Set Enabled >> 'Stepper Number'\")"
        n142 = property on="St1:NewPosition" class="DigNum (strict)"("DisabledEnum"=w331) -> ()  [unwired: 2 in, 2 out]
        n143 = property on="St2:NewPosition" class="DigNum (strict)"("DisabledEnum"=w331) -> ()  [unwired: 2 in, 2 out]
        n144 = property on="St1:Steps" class="DigNum (strict)"("DisabledEnum"=w331) -> ()  [unwired: 2 in, 2 out]
        n145 = property on="St2:Steps" class="DigNum (strict)"("DisabledEnum"=w331) -> ()  [unwired: 2 in, 2 out]
        n146 = property on="St3:NewPosition" class="DigNum (strict)"("DisabledEnum"=w331) -> ()  [unwired: 2 in, 2 out]
        n147 = property on="St3:Steps" class="DigNum (strict)"("DisabledEnum"=w331) -> ()  [unwired: 2 in, 2 out]
        n148 = property on="St1:DoSteps" class="Bool (strict)"("DisabledEnum"=w331) -> ()  [unwired: 2 in, 2 out]
        n149 = call <vilib>:"Add State(s) to Queue__jki_lib_state_machine.vi"("State(s) in (\"\")"=w335) -> ("States Out"=w334:string)  [unwired: 14 in]
      }
      frame "UI: Stepper Fields Set Disabled" {
        w336 = T9."Disabled and Grayed Out" ("Disabled")
        # "Set Stepper Fields state .\n(Usage: \"UI: Stepper Fields Set Enabled >> 'Stepper Number'\")"
        n150 = property on="St1:NewPosition" class="DigNum (strict)"("DisabledEnum"=w336) -> ()  [unwired: 2 in, 2 out]
        n151 = property on="St1:Steps" class="DigNum (strict)"("DisabledEnum"=w336) -> ()  [unwired: 2 in, 2 out]
        n152 = property on="St2:NewPosition" class="DigNum (strict)"("DisabledEnum"=w336) -> ()  [unwired: 2 in, 2 out]
        n153 = property on="St2:Steps" class="DigNum (strict)"("DisabledEnum"=w336) -> ()  [unwired: 2 in, 2 out]
        n154 = property on="St3:NewPosition" class="DigNum (strict)"("DisabledEnum"=w336) -> ()  [unwired: 2 in, 2 out]
        n155 = property on="St3:Steps" class="DigNum (strict)"("DisabledEnum"=w336) -> ()  [unwired: 2 in, 2 out]
        n156 = property on="St1:DoSteps" class="Bool (strict)"("DisabledEnum"=w336) -> ()  [unwired: 2 in, 2 out]
        n157 = call <vilib>:"Add State(s) to Queue__jki_lib_state_machine.vi"("State(s) in (\"\")"=w340) -> ("States Out"=w339:string)  [unwired: 14 in]
      }
      frame "UI: Initialize" {
        n158 = call <vilib>:"Add State(s) to Queue__jki_lib_state_machine.vi"("State(s) in Front (\"\")"="UI: Stepper Fields Set Enabled" ("State(s) in Front (\"\")"), "State(s) in (\"\")"=w345) -> ("States Out"=w344:string)  [unwired: 13 in]
      }
      frame "UI: Steps to new position" {
        n159 = case shown="\"3\"" w346 {
          frame "1" {
            n160 = local read "St1:Position"() -> (w352:dbl)
            n161 = local read "St1:Steps"() -> (w351:dbl)
            n162 = Add(x=w352, y=w351) -> (x+y=w350:dbl)
            n163 = local write "St1:NewPosition"(w350) -> ()
          }
          frame "2" {
            n164 = local read "St2:Position"() -> (w355:dbl)
            n165 = local read "St2:Steps"() -> (w354:dbl)
            n166 = Add(x=w355, y=w354) -> (x+y=w353:dbl)
            n167 = local write "St2:NewPosition"(w353) -> ()
          }
          frame "3" {
            n168 = local read "St3:Position"() -> (w358:dbl)
            n169 = local read "St3:Steps"() -> (w357:dbl)
            n170 = Add(x=w358, y=w357) -> (x+y=w356:dbl)
            n171 = local write "St3:NewPosition"(w356) -> ()
          }
          frame Default {
          }
        }
      }
      frame "UI: New WL to positions" {
        n172 = local read "WL:WLToStepper1"() -> (w365:dbl[][])
        n173 = local read "WL:WLToStepper2"() -> (w363:dbl[][])
        n174 = local read "WL:WLToStepper3"() -> (w364:dbl[][])
        n175 = property on="WL:NewValue" class="DigNum (strict)"() -> ("Value"=w359:dbl)  [unwired: 2 in, 2 out]
        n176 = call "GetNearestValue.vi"("Value"=w359, "Array"=w365) -> ("Nearest Value"=w362:dbl)  [unwired: 9 in]
        n177 = call "GetNearestValue.vi"("Value"=w359, "Array"=w363) -> ("Nearest Value"=w361:dbl)  [unwired: 9 in]
        n178 = call "GetNearestValue.vi"("Value"=w359, "Array"=w364) -> ("Nearest Value"=w360:dbl)  [unwired: 9 in]
        n179 = property on="St1:NewPosition" class="DigNum (strict)"("Val(Sgnl)"=w362) -> ()  [unwired: 2 in, 2 out]
        n180 = property on="St2:NewPosition" class="DigNum (strict)"("Val(Sgnl)"=w361) -> ()  [unwired: 2 in, 2 out]
        n181 = property on="St3:NewPosition" class="DigNum (strict)"("Val(Sgnl)"=w360) -> ()  [unwired: 2 in, 2 out]
      }
      frame "UI: New position to steps" {
        n182 = case shown="Default" w370 {
          frame Default {
          }
          frame "1" {
            n183 = local read "St1:NewPosition"() -> (w375:dbl)
            n184 = local read "St1:Position"() -> (w374:dbl)
            n185 = Subtract(x=w375, y=w374) -> (x-y=w373:dbl)
            n186 = local write "St1:Steps"(w373) -> ()
          }
          frame "2" {
            n187 = local read "St2:NewPosition"() -> (w378:dbl)
            n188 = local read "St2:Position"() -> (w377:dbl)
            n189 = Subtract(x=w378, y=w377) -> (x-y=w376:dbl)
            n190 = local write "St2:Steps"(w376) -> ()
          }
          frame "3" {
            n191 = local read "St3:NewPosition"() -> (w381:dbl)
            n192 = local read "St3:Position"() -> (w380:dbl)
            n193 = Subtract(x=w381, y=w380) -> (x-y=w379:dbl)
            n194 = local write "St3:Steps"(w379) -> ()
          }
        }
      }
      frame "UI: Cursor Set" {
        # "Set and Unset Cursor Busy.\n(Usage: \"UI: Cursor Set >> Busy|Idle\")"
        n195 = call <vilib>:"Add State(s) to Queue__jki_lib_state_machine.vi"("State(s) in (\"\")"=w385) -> ("States Out"=w384:string)  [unwired: 14 in]
      }
      frame "UI: RefreshLED Set" {
        # "Argument"
        # "Set and Unset RefreshLED.\n(Usage: \"UI: RefreshLED Set >> On|Off\")"
        n196 = case shown="\"Off\", Default" w389 {
          tunnel: [TRUE FALSE] -> w387
          frame "On" {
          }
          frame "Off", Default {
          }
        }
        "App:RefreshLED" <- w387
      }
      frame "UI: Front Panel State" {
        # "Set Front Panel Open or Closed\n(Usage: \"UI: Front Panel State >> Open|Close\")"
      }
      frame "---------- Macro ----------" {
        # "Do not put any code in this frame.\n(It is a separator no-op. You can make a copy of this frame to create a new Macro frame)"
        n197 = call <vilib>:"Add State(s) to Queue__jki_lib_state_machine.vi"("State(s) in (\"\")"=w399) -> ("States Out"=w398:string)  [unwired: 14 in]
      }
      frame "Macro: Initialize" {
        w400 = "Data: Initialize\nInitialize Core Data\nUI: Initialize\nUI: Front Panel State >> Open\nData: Load Conversion Files\nData: Read Config\nSteppers: Connect"  # Data: Initialize Initialize Core Data UI: Initialize UI: Front Panel State >> Open Data: Load Conversion Files Data: Read Config Steppers: Connect
        # "Initialization Macro\n(This is called once, when the VI starts)"
        n198 = call <vilib>:"Add State(s) to Queue__jki_lib_state_machine.vi"("State(s) in Front (\"\")"=w400, "State(s) in (\"\")"=w404) -> ("States Out"=w403:string)  [unwired: 13 in]
      }
      frame "Macro: Refresh" {
        n199 = Unbundle By Name(w407) -> ("isConnected"=w406:bool)
        n200 = case shown="True" w406 {
          tunnel: ["" "UI: RefreshLED Set >> On\nSteppers: Refresh\nSteppers: Refresh WL\nUI: RefreshLED Set >> Off\nData: Write Config"] -> w405
          frame False {
          }
          frame True {
          }
        }
        n201 = call <vilib>:"Add State(s) to Queue__jki_lib_state_machine.vi"("State(s) in Front (\"\")"=w405, "State(s) in (\"\")"=w410) -> ("States Out"=w409:string)  [unwired: 13 in]
      }
      frame "Macro: Exit" {
        # "Exit Macro\n(This is called once, when the VI exits)"
        n202 = Unbundle By Name(w419) -> ("Core.Close Panel on Exit?"=w418:bool)
        n203 = Select(t="UI: Front Panel State >> Close", s=w418, f="") -> (s? t:f=w415:string)
        n204 = call <vilib>:"Add State(s) to Queue__jki_lib_state_machine.vi"("State(s) in (\"\")"=w415, "State(s) at Back (\"\")"="Steppers: Disconnect\nData: Cleanup\nExit") -> ("States Out"=w413:string)  [unwired: 13 in]
        n205 = call <vilib>:"Add State(s) to Queue__jki_lib_state_machine.vi"("State(s) in Front (\"\")"=w413, "State(s) in (\"\")"=w422) -> ("States Out"=w421:string)  [unwired: 13 in]
      }
      frame "---------- Steppers ----------" {
        # "Template Separator\n(You can make a copy of, or modify, this frame)"
        n206 = call <vilib>:"Add State(s) to Queue__jki_lib_state_machine.vi"("State(s) in (\"\")"=w426) -> ("States Out"=w425:string)  [unwired: 14 in]
      }
      frame "Steppers: Connect" {
        # "Connect to steppers"
        n207 = call "connect.vi"("error in"=w428, "VISA resource name"="App:ResourceName") -> ("error out"=w427:errorcluster, "VISA resource name out"=w430:refnum<visa-resource-name>)
        n208 = Unbundle By Name(w427) -> ("status"=w429:bool)
        n209 = Not(x=w429) -> (.not. x?=w432:bool)
        n210 = Bundle By Name(cluster=w437, "isConnected"=w432, "VISA resource"=w430) -> (w436:T5)
        n211 = call <vilib>:"Add State(s) to Queue__jki_lib_state_machine.vi"("State(s) in Front (\"\")"="Macro: Refresh\nSteppers: Set position >> 1\nSteppers: Set position >> 2\nSteppers: Set position >> 3" ("State(s) at Back (\"\")"), "State(s) in (\"\")"=w434) -> ("States Out"=w435:string)  [unwired: 13 in]
      }
      frame "Steppers: Disconnect" {
        n212 = Unbundle By Name(w440) -> ("VISA resource"=w444:refnum<visa-resource-name>)
        n213 = call "disconnect.vi"("error in"=w443, "VISA resource name"=w444) -> ("error out"=w442:errorcluster)  [unwired: 1 in]
        n214 = Bundle By Name(cluster=w440, "isConnected"=FALSE) -> (w439:T5)
      }
      frame "Steppers: Do steps" {
        w451 = ""
        n215 = case shown="Default" w450 {
          tunnel: [0.0 ("St3:NewPosition") w462 w463 w464] -> w452
          frame Default {
          }
          frame "1" {
            n216 = local read "St1:NewPosition"() -> (w462:dbl)
          }
          frame "2" {
            n217 = local read "St2:NewPosition"() -> (w463:dbl)
          }
          frame "3" {
            n218 = local read "St3:NewPosition"() -> (w464:dbl)
          }
        }
        n219 = Decimal String To Number(string=w450) -> (number=w449:i32)  [unwired: 2 in, 1 out]
        n220 = Decrement(x=w449) -> (x-1=w448:i32)
        n221 = Unbundle By Name(w458) -> ("VISA resource"=w457:refnum<visa-resource-name>)
        n222 = Number To Fractional String(use system decimal point (T)=FALSE, number=w452) -> (F-format string=w447:string)  [unwired: 2 in]
        n223 = Build Array(w451, w451, w451) -> (w446:string[])
        n224 = Insert Into Array(array=w446, index=w448, new element=w447) -> (w445:string[])
        n225 = call "MoveTo.vi"("error in (no error)"=w456, "speed"="Speed", "positions"=w445, "VISA Refnum in"=w457) -> ("error out"=w455:errorcluster)  [unwired: 6 in, 1 out]
        n226 = call <vilib>:"Add State(s) to Queue__jki_lib_state_machine.vi"("State(s) in (\"\")"=w460) -> ("States Out"=w459:string)  [unwired: 14 in]
      }
      frame "Steppers: Set All" {
        n227 = local read "St1:NewPosition"() -> (w470:dbl)
        n228 = local read "St2:NewPosition"() -> (w469:dbl)
        n229 = local read "St3:NewPosition"() -> (w468:dbl)
        n230 = Unbundle By Name(w475) -> ("VISA resource"=w474:refnum<visa-resource-name>)
        n231 = Build Array(w470, w469, w468) -> (w467:dbl[])
        n232 = Number To Fractional String(use system decimal point (T)=FALSE, number=w467) -> (F-format string=w466:string[])  [unwired: 2 in]
        n233 = local read "Speed"() -> (w465:string)
        n234 = call "MoveTo.vi"("error in (no error)"=w473, "speed"=w465, "positions"=w466, "VISA Refnum in"=w474) -> ("error out"=w472:errorcluster)  [unwired: 6 in, 1 out]
        n235 = call <vilib>:"Add State(s) to Queue__jki_lib_state_machine.vi"("State(s) in (\"\")"=w477) -> ("States Out"=w476:string)  [unwired: 14 in]
      }
      frame "Steppers: Set position" {
        w486 = ""
        n236 = case shown="\"1\"" w490 {
          tunnel: [0 ("St3:Steps") w496 w497 w498] -> w480
          frame Default {
          }
          frame "1" {
            n237 = local read "St1:NewPosition"() -> (w496:dbl)
          }
          frame "2" {
            n238 = local read "St2:NewPosition"() -> (w497:dbl)
          }
          frame "3" {
            n239 = local read "St3:NewPosition"() -> (w498:dbl)
          }
        }
        n240 = Decimal String To Number(string=w490, default (0L)=u16 0 ("default (0 I32)")) -> (number=w484:u16)  [unwired: 1 in, 1 out]
        n241 = Decrement(x=w484) -> (x-1=w483:u16)
        n242 = Build Array(w486, w486, w486) -> (w485:string[])
        n243 = Unbundle By Name(w491) -> ("VISA resource"=w487:refnum<visa-resource-name>)
        n244 = Number To Fractional String(use system decimal point (T)=FALSE, number=w480) -> (F-format string=w478:string)  [unwired: 2 in]
        n245 = Replace Array Subset(array=w485, new element=w478, index=w483) -> (w482:string[])
        n246 = call "SetPosition.vi"("error in (no error)"=w488, "positions"=w482, "VISA Refnum in"=w487) -> ("error out"=w489:errorcluster)  [unwired: 7 in, 1 out]
        n247 = call <vilib>:"Add State(s) to Queue__jki_lib_state_machine.vi"("State(s) in (\"\")"=w494, "State(s) at Back (\"\")"="Data: Write Config" ("State(s) at Back (\"\")")) -> ("States Out"=w493:string)  [unwired: 13 in]
      }
      frame "Steppers: Stop" {
        n248 = Unbundle By Name(w503) -> ("VISA resource"=w502:refnum<visa-resource-name>)
        n249 = call "Stop.vi"("error in (no error)"=w501, "VISA Refnum in"=w502) -> ("error out"=w500:errorcluster)  [unwired: 8 in, 1 out]
        n250 = call <vilib>:"Add State(s) to Queue__jki_lib_state_machine.vi"("State(s) in (\"\")"=w505, "State(s) at Back (\"\")"="Data: Write Config" ("State(s) at Back (\"\")")) -> ("States Out"=w504:string)  [unwired: 13 in]
      }
      frame "Steppers: Refresh" {
        n251 = Unbundle By Name(w513) -> ("VISA resource"=w512:refnum<visa-resource-name>, "isConnected"=w509:bool)
        n252 = case shown="True" w509 {
          tunnel: w512 -> [_ w519]
          tunnel: w511 -> [w514 w520]
          tunnel: [w514 w521] -> w510
          frame False {
          }
          frame True {
            n253 = call "GetCurrentStatus.vi"("error in (no error)"=w520, "VISA Refnum in"=w519) -> ("error out"=w521:errorcluster, "status"=w522:T10)  [unwired: 7 in, 1 out]
            n254 = Unbundle By Name(w522) -> ("current"=w523:dbl[], "boundaries"=w518:T4[], "is running"=w515:bool)
            n255 = case shown="False" w515 {
              frame False {
                n256 = property on="St:Stop" class="Bool (strict)"("Val(Sgnl)"=TRUE) -> ()  [unwired: 2 in, 2 out]
              }
              frame True {
              }
            }
            n257 = for {
              tunnel: w523 -> [w530] mode=indexing
              tunnel: w518 -> [w527] mode=indexing
              tunnel: BoundaryStatus."NO BOUNDARY" ("Enum") -> [w525]
              tunnel: BoundaryStatus."OUT OF LEFT" ("Enum") -> [w528]
              i -> [w532]
              n258 = Not Equal?(x=w527, y=w525) -> (x != y?=w529:bool)
              n259 = Increment(x=w532) -> (x+1=w531:i32)
              n260 = Equal?(x=w527, y=w528) -> (x = y?=w526:bool)
              n261 = case shown="3" w531 {
                tunnel: w530 -> [_ w537 w550 w563]
                tunnel: w527 -> [_ _ _ _]
                tunnel: w529 -> [_ w536 w549 w562]
                tunnel: w526 -> [_ w535 w548 w561]
                frame Default {
                }
                frame 1 {
                  n262 = case shown="True" w536 {
                    tunnel: w535 -> [_ w541]
                    tunnel: [w538 w540] -> w534
                    tunnel: [w538 w539] -> w533
                    frame False {
                      w538 = FALSE
                    }
                    frame True {
                      n263 = case shown="False" w541 {
                        tunnel: [FALSE TRUE] -> w540
                        tunnel: [TRUE FALSE] -> w539
                        frame False {
                        }
                        frame True {
                        }
                      }
                    }
                  }
                  "St1:Right" <- w533
                  "St1:Left" <- w534
                  "St1:Position" <- w537
                }
                frame 2 {
                  n264 = case shown="False" w549 {
                    tunnel: w548 -> [_ w554]
                    tunnel: [w551 w553] -> w547
                    tunnel: [w551 w552] -> w546
                    frame False {
                      w551 = FALSE
                    }
                    frame True {
                      n265 = case shown="False" w554 {
                        tunnel: [FALSE TRUE] -> w553
                        tunnel: [TRUE FALSE] -> w552
                        frame False {
                        }
                        frame True {
                        }
                      }
                    }
                  }
                  "St2:Left" <- w547
                  "St2:Right" <- w546
                  "St2:Position" <- w550
                }
                frame 3 {
                  n266 = case shown="True" w562 {
                    tunnel: w561 -> [_ w567]
                    tunnel: [w564 w566] -> w559
                    tunnel: [w564 w565] -> w560
                    frame False {
                      w564 = FALSE
                    }
                    frame True {
                      n267 = case shown="True" w567 {
                        tunnel: [FALSE TRUE] -> w566
                        tunnel: [TRUE FALSE] -> w565
                        frame False {
                        }
                        frame True {
                        }
                      }
                    }
                  }
                  "St3:Left" <- w559
                  "St3:Right" <- w560
                  "St3:Position" <- w563
                }
              }
            }
          }
        }
        n268 = call <vilib>:"Add State(s) to Queue__jki_lib_state_machine.vi"("State(s) in Front (\"\")"="UI: New position to steps >> 1\nUI: New position to steps >> 2\nUI: New position to steps >> 3\nData: Write Config" ("State(s) at Back (\"\")"), "State(s) in (\"\")"=w508) -> ("States Out"=w507:string)  [unwired: 13 in]
      }
      frame "Steppers: Refresh WL" {
        n269 = call-dynamic "Get Parameter.vi"("error in (no error)"=w573, "Stepper3D in"=w574) -> ("error out"=w572:errorcluster)  [unwired: 7 in, 2 out]
        n270 = call <vilib>:"Add State(s) to Queue__jki_lib_state_machine.vi"("State(s) in (\"\")"=w576) -> ("States Out"=w575:string)  [unwired: 14 in]
      }
      frame "---------- Utils ---------" {
        # "Template Separator\n(You can make a copy of, or modify, this frame)"
        n271 = call <vilib>:"Add State(s) to Queue__jki_lib_state_machine.vi"("State(s) in (\"\")"=w581) -> ("States Out"=w580:string)  [unwired: 14 in]
      }
      frame "Utils: Wait ms" {
        # "Wait ms >> \"number of ms\""
        n272 = Decimal String To Number(string=w584, default (0L)=u32 0 ("default (0 I32)")) -> (number=w583:u32)  [unwired: 1 in, 1 out]
        n273 = Wait (ms)(milliseconds to wait=w583) -> ()  [unwired: 1 out]
        n274 = call <vilib>:"Add State(s) to Queue__jki_lib_state_machine.vi"("State(s) in (\"\")"=w588) -> ("States Out"=w587:string)  [unwired: 14 in]
      }
    }
  }
  n275 = call-parent "Actor Core.vi"("error in"=w14, "Actor in"=w15) -> ("error out"=w13:errorcluster, "Actor out"=w12:refnum<class "Actor.lvclass">)  [unwired: 8 in]
  n276 = call "Destroy Observer.vi"("observer in"=w4) -> ()  [unwired: 11 in]
  n277 = call "Send Last Stop Event.vi"("error in (no error)"=w13, "Actor in"=w12) -> ("error out"=→"error out":errorcluster, "Actor  out"=→"Actor  out":refnum<class "Actor.lvclass">)  [unwired: 8 in]
  "Stop" <- FALSE ("Stop")
